vi "Convert Runtime Cluster to JSON Cluster.vi"(8 "error in (no error)":errorcluster, 11 "Framework Configuration":T1) -> (0 "error out":errorcluster, 3 "Framework JSON Configuration":T13)   [LabVIEW 2017, in "DSF Core.lvlib" / "Configuration Session.lvclass"]
uses:
  Configuration Session.lvclass
  Typedefs/DSF File Format 1.0 Framework v1.ctl
  Typedefs/DSF File Format 1.0 Plugin.ctl
  Typedefs/DSF Timing Info.ctl
  Typedefs/DSF Engine Plugin Thread Configuration.ctl
  Typedefs/DSF Settings Info.ctl
  Typedefs/DSF File Format 1.0 Transfer Group.ctl
  Typedefs/DSF File Format 1.0 Transfer.ctl
  Typedefs/DSF File Format 1.0 Channel.ctl
  Typedefs/DSF Engine Framework Configuration.ctl
  Typedefs/DSF Engine Plugin Configuration.ctl
  Typedefs/DSF Engine Transfer Group Configuration.ctl
  Typedefs/DSF Direction.ctl
  Typedefs/DSF Engine Transfer Configuration.ctl
  Typedefs/DSF Byte Order.ctl
  Typedefs/DSF Engine Channel Configuration.ctl
  Typedefs/DSF Data Type.ctl
  Typedefs/DSF Timeout Behavior.ctl
  DSF Core.lvlib
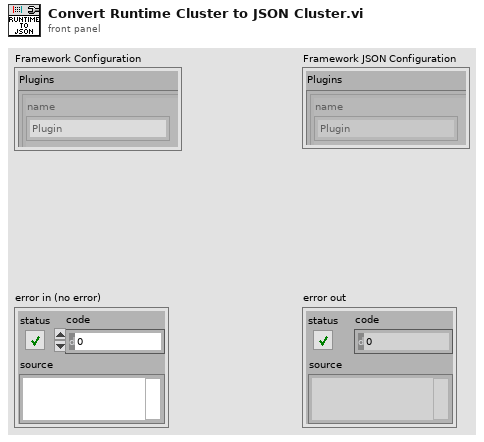
[diagram p1: front panel]
types:
  T1 = typedef "DSF Core.lvlib/DSF Engine Framework Configuration.ctl" = cluster{"Plugins":T2[]}
  T2 = typedef "DSF Core.lvlib/DSF Engine Plugin Configuration.ctl" = cluster{"name":string, "components":string[], "cycle timing":T3, "threads":T4[], "Transfer Groups":T6[], "settings":T5}
  T3 = typedef "DSF Core.lvlib/DSF Timing Info.ctl" = cluster{"priority":u64, "decimation":u64, "offset":u64}
  T4 = typedef "DSF Core.lvlib/DSF Engine Plugin Thread Configuration.ctl" = cluster{"buffer converter settings":T5, "transceiver settings":T5, "custom settings":T5, "processor":i32, "priority offset":i16}
  T5 = typedef "DSF Core.lvlib/DSF Settings Info.ctl" = cluster{"key":string, "value":string}[]
  T6 = typedef "DSF Core.lvlib/DSF Engine Transfer Group Configuration.ctl" = cluster{"name":string, "direction":T7, "cycle timing":T3, "thread index":i32, "settings":T5, "Transfers":T8[], "timeout behavior":T12}
  T7 = typedef "DSF Core.lvlib/DSF Direction.ctl" = enum8{"Tx", "Rx"}
  T8 = typedef "DSF Core.lvlib/DSF Engine Transfer Configuration.ctl" = cluster{"name":string, "byte order":T9, "settings":T5, "channels":T10[]}
  T9 = typedef "DSF Core.lvlib/DSF Byte Order.ctl" = enum8{"big-endian", "little-endian"}
  T10 = typedef "DSF Core.lvlib/DSF Engine Channel Configuration.ctl" = cluster{"string offset":u64, "string data type":T11, "engine data type":T11, "name":string, "settings":T5, "units":string}
  T11 = typedef "DSF Core.lvlib/DSF Data Type.ctl" = enum8{"Bool", "SGL", "DBL", "I8", "I16", "I32", "I64", "U8", "U16", "U32", "U64"}
  T12 = typedef "DSF Core.lvlib/DSF Timeout Behavior.ctl" = enum8{"Increment Late Count", "Throw Error"}
  T13 = typedef "DSF Core.lvlib/Configuration Session.lvclass/DSF File Format 1.0 Framework v1.ctl" = cluster{"Plugins":T14[]}
  T14 = typedef "DSF Core.lvlib/Configuration Session.lvclass/DSF File Format 1.0 Plugin.ctl" = cluster{"name":string, "components":string[], "cycle timing":T3, "threads":T4[], "Transfer Groups":T15[], "settings":T5}
  T15 = typedef "DSF Core.lvlib/Configuration Session.lvclass/DSF File Format 1.0 Transfer Group.ctl" = cluster{"name":string, "direction":u8, "cycle timing":T3, "thread index":i32, "settings":T5, "Transfers":T16[], "timeout behavior":u8}
  T16 = typedef "DSF Core.lvlib/Configuration Session.lvclass/DSF File Format 1.0 Transfer.ctl" = cluster{"name":string, "byte order":u8, "settings":T5, "channels":T17[]}
  T17 = typedef "DSF Core.lvlib/Configuration Session.lvclass/DSF File Format 1.0 Channel.ctl" = cluster{"string offset":u64, "string data type":u8, "engine data type":u8, "name":string, "settings":T5, "units":string}
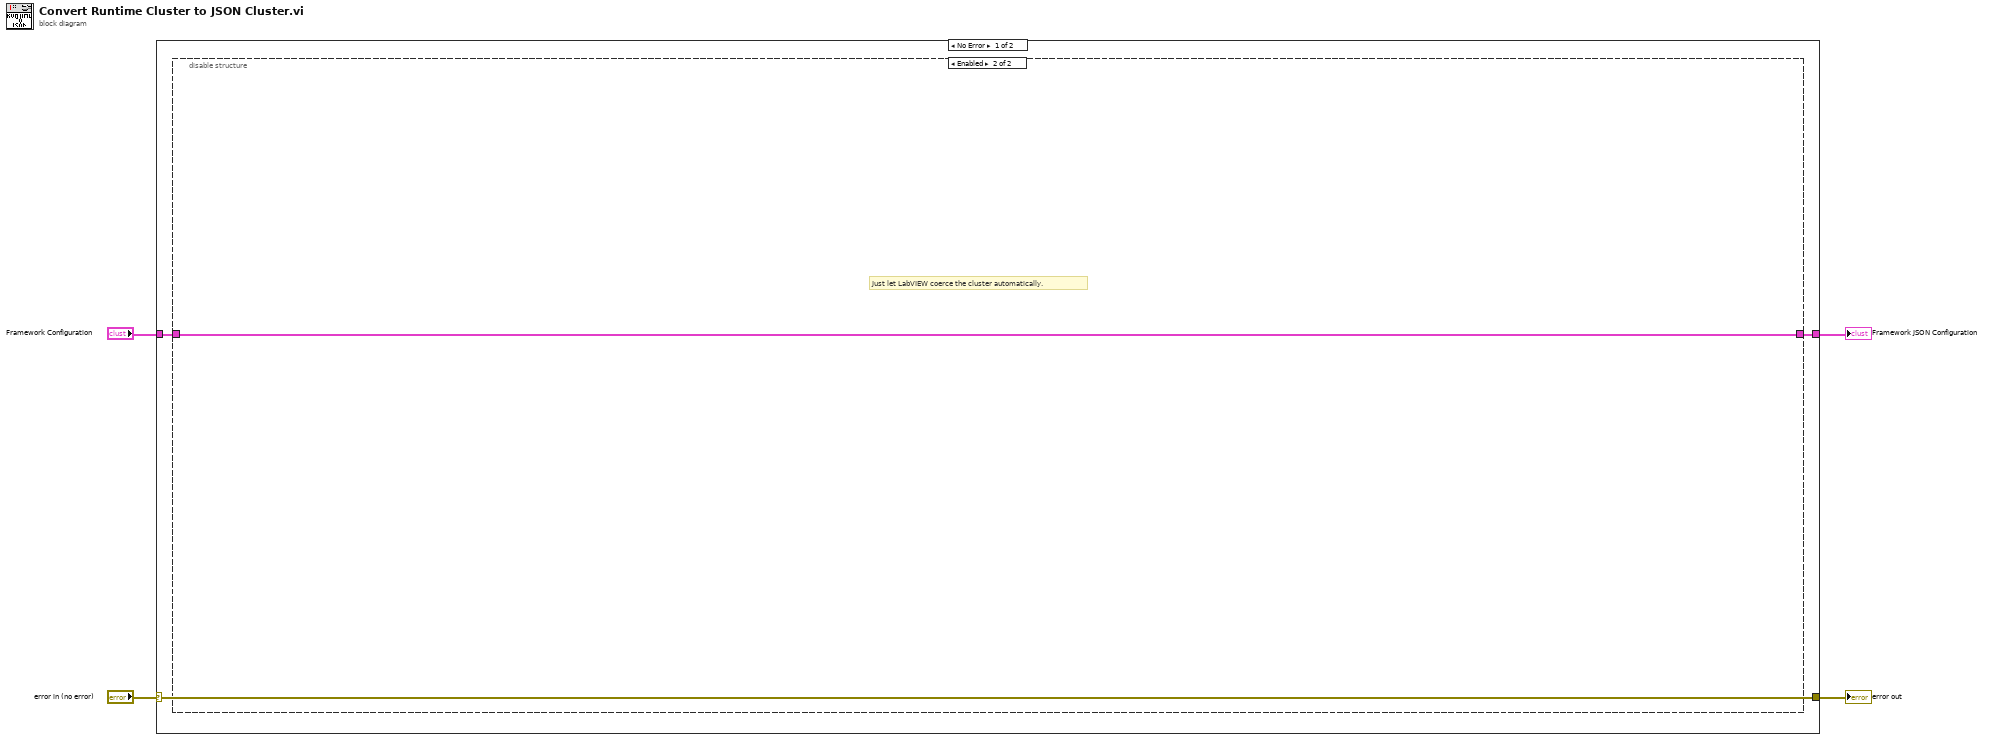
[diagram p0: block diagram]
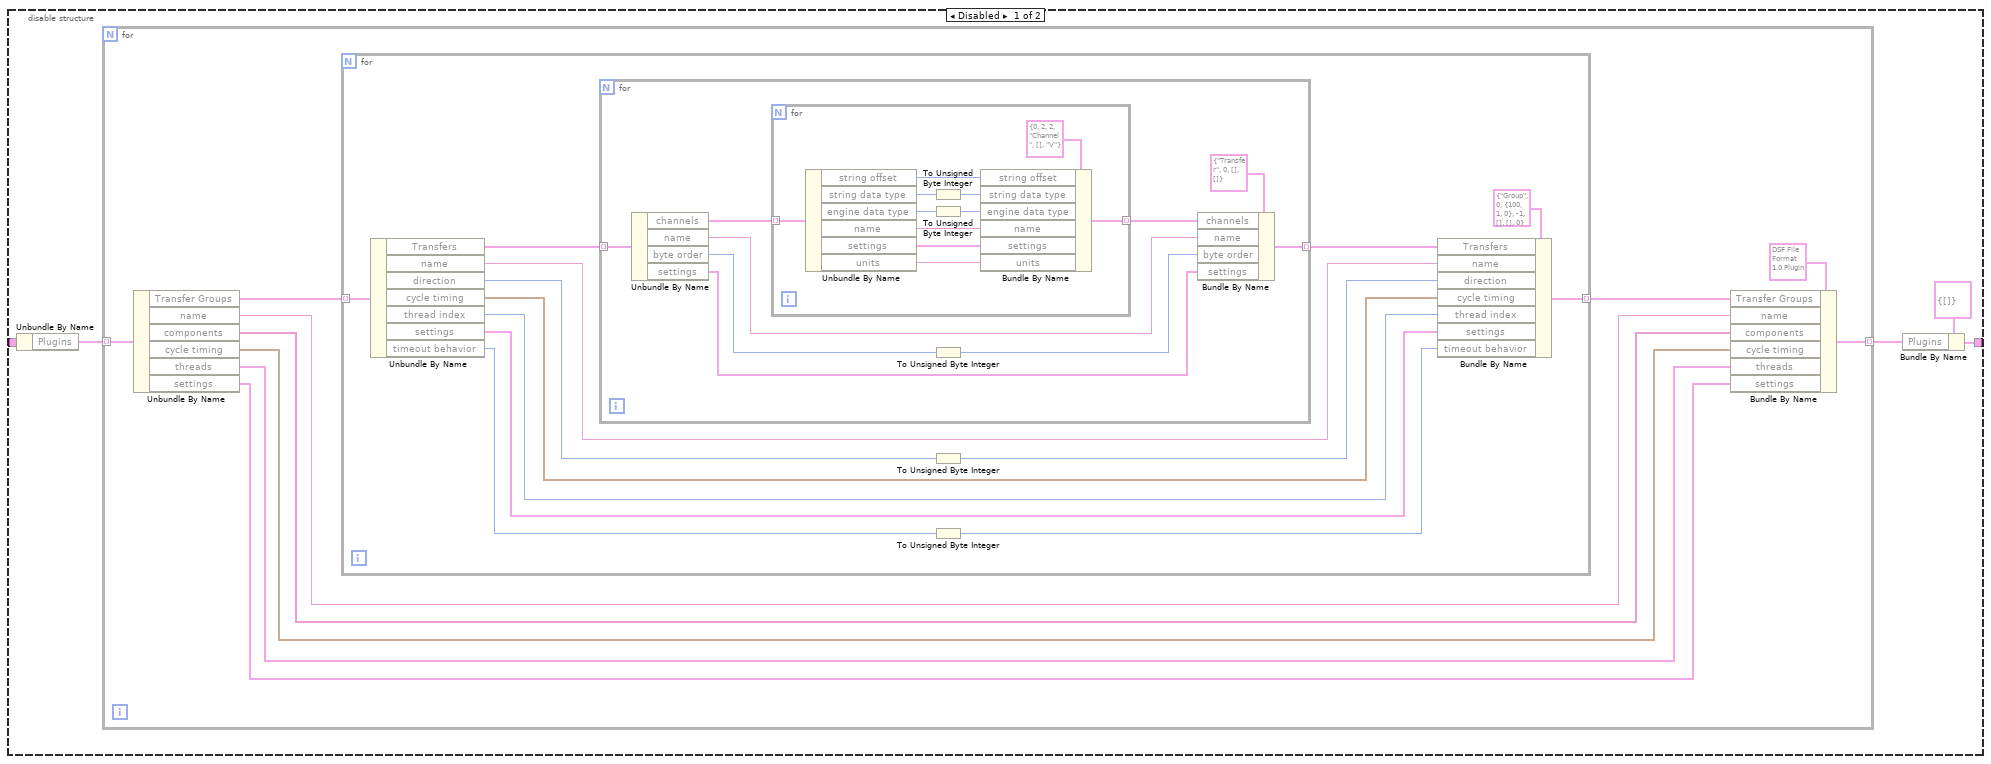
[diagram p2: hidden frame]
diagram:
  n1 = case shown="No Error" "error in (no error)" {
    selector: "error in (no error)" -> [w5 w57]
    tunnel: [w7 _] -> w4
    tunnel: "Framework Configuration" -> [w6 _]
    tunnel: [w5 w57] -> w1
    frame No Error {
      n2 = disable-structure shown="Enabled" {
        disable-tunnel: [w10 w56] -> w7
        disable-tunnel: w6 -> [w8 w56]
        frame Disabled {
          n3 = Unbundle By Name(w8) -> ("Plugins"=w11:T2[])
          n4 = for {
            tunnel: w11 -> [w22] mode=indexing
            tunnel: [w13] -> w12 mode=indexing
            n5 = Unbundle By Name(w22) -> ("Transfer Groups"=w21:T6[], "name"=w14:string, "components"=w18:string[], "cycle timing"=w17:T3, "threads"=w16:T4[], "settings"=w15:T5)
            n6 = for {
              tunnel: w21 -> [w35] mode=indexing
              tunnel: [w23] -> w19 mode=indexing
              n7 = Unbundle By Name(w35) -> ("Transfers"=w34:T8[], "name"=w31:string, "direction"=w30:T7, "cycle timing"=w28:T3, "thread index"=w27:i32, "settings"=w26:T5, "timeout behavior"=w25:T12)
              n8 = for {
                tunnel: w34 -> [w44] mode=indexing
                tunnel: [w36] -> w32 mode=indexing
                n9 = Unbundle By Name(w44) -> ("channels"=w43:T10[], "name"=w40:string, "byte order"=w39:T9, "settings"=w38:T5)
                n10 = for {
                  tunnel: w43 -> [w55] mode=indexing
                  tunnel: [w45] -> w41 mode=indexing
                  n11 = Unbundle By Name(w55) -> ("string offset"=w48:u64, "string data type"=w49:T11, "engine data type"=w50:T11, "name"=w51:string, "settings"=w52:T5, "units"=w53:string)
                  n12 = To Unsigned Byte Integer(number=w49) -> (unsigned 8bit integer=w46:u8)
                  n13 = To Unsigned Byte Integer(number=w50) -> (unsigned 8bit integer=w47:u8)
                  n14 = Bundle By Name(cluster=T17 {"string offset"=0, "string data type"=2, "engine data type"=2, "name"="Channel", "settings"=[], "units"="V"} ("channel configuration"), "string offset"=w48, "string data type"=w46, "engine data type"=w47, "name"=w51, "settings"=w52, "units"=w53) -> (w45:T17)
                }
                n15 = To Unsigned Byte Integer(number=w39) -> (unsigned 8bit integer=w37:u8)
                n16 = Bundle By Name(cluster=T16 {"name"="Transfer", "byte order"=0, "settings"=[], "channels"=[]} ("Transfer Configuration"), "channels"=w41, "name"=w40, "byte order"=w37, "settings"=w38) -> (w36:T16)
              }
              n17 = To Unsigned Byte Integer(number=w30) -> (unsigned 8bit integer=w29:u8)
              n18 = To Unsigned Byte Integer(number=w25) -> (unsigned 8bit integer=w24:u8)
              n19 = Bundle By Name(cluster=T15 {"name"="Group", "direction"=0, "cycle timing"={"priority"=100, "decimation"=1, "offset"=0}, "thread index"=-1, "settings"=[], "Transfers"=[], "timeout behavior"=0} ("Transfer Group Configuration"), "Transfers"=w32, "name"=w31, "direction"=w29, "cycle timing"=w28, "thread index"=w27, "settings"=w26, "timeout behavior"=w24) -> (w23:T15)
            }
            n20 = Bundle By Name(cluster=T14 {"name"="Plugin", "components"=[], "cycle timing"={"priority"=10000, "decimation"=1, "offset"=0}, "threads"=[], "Transfer Groups"=[], "settings"=[]} ("Plugin Configuration"), "Transfer Groups"=w19, "name"=w14, "components"=w18, "cycle timing"=w17, "threads"=w16, "settings"=w15) -> (w13:T14)
          }
          n21 = Bundle By Name(cluster=T13 {"Plugins"=[]} ("Framework Configuration"), "Plugins"=w12) -> (w10:T13)
        }
        frame Enabled {
          # "Just let LabVIEW coerce the cluster automatically."
        }
      }
    }
    frame Error {
    }
  }
  "Framework JSON Configuration" <- w4
  "error out" <- w1
